vi "DAT to LV.vi"(8 "header length":i32=11, 11 "File Path":path=path "\\\\tiles\\Data/SA02777G.graphene.20150414/12 - sweep B +-2T, step Vsg/SA02777G.graphene.20150414.000000.dat") -> (1 "Comments":string="sweep Vsg (22): 750mV to -500mV 50mV steps\r\n\r\n\r\n\r\n\r\n\r\n\r\n\r\n\r\n\r\n\r\n\r\n\r\n\r\n\r\nB=0T to 2T to -2T to 0T, 0.0104 A/s\r\n\r\n\r\n\r\n\r\n\r\n\r\n\r\n\r\n\r\n\r\n\r\n\r\n\r\n\r\n\r\n\r\n\r\n\r\n\r\n\r\n\r\n\r\n\r\n\r\n\r\n\r\n\r\n\r\n\r\nlockin\r\n\r\n\r\n\r\n\r\n\r\n\r\n\r\n\r\n\r\n\r\n\r\n\r\n\r\n\r\n0: 1\r\n\r\n\r\n\r\n\r\n\r\n\r\n\r\n\r\n\r\n\r\n\r\n\r\n\r\n\r\n1: 3\r\n\r\n\r\n\r\n\r\n\r\n\r\n\r\n\r\n\r\n\r\n\r\n\r\n\r\n\r\n2: 4, current\r\n\r\n\r\n\r\n\r\n\r\n\r\n\r\n\r\n\r\n\r\n\r\n\r\n\r\n\r\n3: 5\r\n\r\n\r\n\r\n\r\n\r\n\r\n\r\n\r\n\r\n\r\n\r\n\r\n\r\n\r\n4: 27\r\n\r\n\r\n\r\n\r\n\r\n\r\n\r\n\r\n\r\n\r\n\r\n\r\n\r\n\r\n5: 28, current, 8mV AC\r\n\r\n\r\n\r\n\r\n\r\n\r\n\r\n\r\n\r\n\r\n\r\n\r\n\r\n\r\nappliedVsg= 0.750000\r\n\r\n\r\n\r\n\r\n\r\n\r\n\r\n\r\n\r\n\r\n\r\n\r\n\r\n\r\n", 2 "Wavenames":string[](array[string])=["time", "temp", "Bfield", "X0", "Y0", "X1", "Y1", "X2", "Y2", "X3", "Y3", "X4", "Y4", "X5", "Y5"], 3 "Data":dbl[][](array[numeric]))   [LabVIEW 2013]
uses:
  <vilib>/Utility/file.llb/Read From Spreadsheet File (string).vi
panel:
  out "all rows":string[][](array[string])
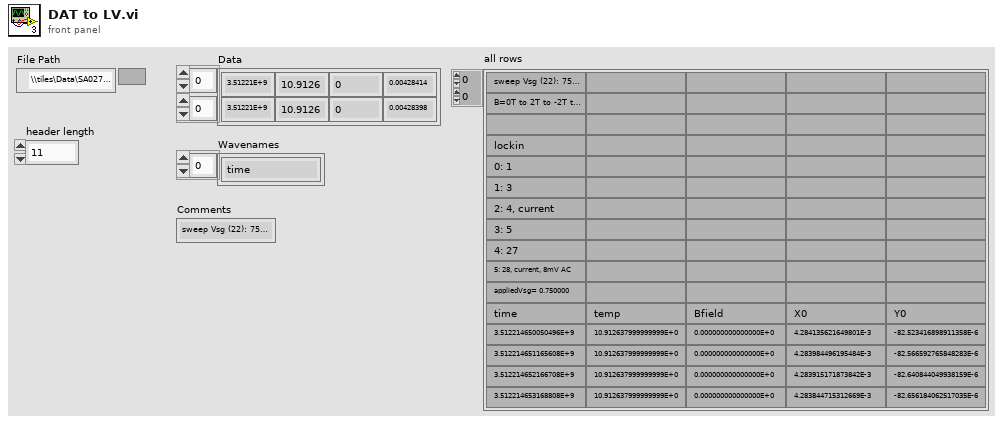
[diagram p1: front panel]
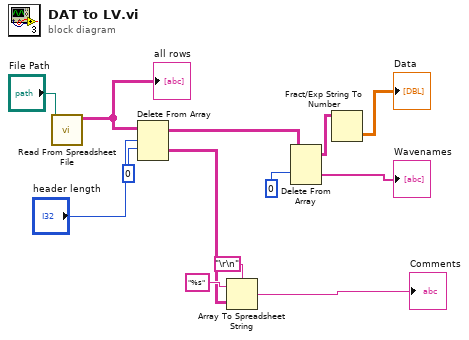
[diagram p0: block diagram]
diagram:
  n1 = call-poly <vilib>:"Read From Spreadsheet File.vi"("file path (dialog if empty)"="File Path") -> ("all rows"=w3:string[][])  [unwired: 6 in, 4 out]
  "all rows" <- w3
  n2 = Delete From Array(array=w3, length="header length", index (row)=0) -> (deleted portion=w5:string[][], array with subset deleted=w9:string[][])  [unwired: 1 in]
  n3 = Array To Spreadsheet String(delimiter (Tab)="\r\n", array=w5, 3:"%s" ("format string")) -> (spreadsheet string=→"Comments":string)
  n4 = Delete From Array(array=w9, index (row)=0) -> (deleted portion=→"Wavenames":string[], array with subset deleted=w11:string[][])  [unwired: 2 in]
  n5 = Fract/Exp String To Number(string=w11) -> (number=→"Data":dbl[][])  [unwired: 3 in, 1 out]
